vi "Display.vi"(8 "error in":errorcluster, 11 "Input (String) in":refnum<class "Custom - Input (String).lvclass">) -> (0 "error out":errorcluster, 3 "Input (String) out":refnum<class "Custom - Input (String).lvclass">)   [LabVIEW 2021, in "Pop-Up.lvlib" / "Custom - Input (String).lvclass"]
doc: "This vi will display the input pop up waiting for a type string input from the user while displaying a custom graphic to the user.\n\n<b>Code Developed By:</b> +\nDaniel Coons +\nhttps://github.com/danielcoons/tsc-pop-up"
uses:
  Custom - Input (String).lvclass
  C:/Development/Open Source/tsc-pop-up/Popup/Popup.lvclass
  Custom - Input (String).lvclass/Custom - Input (String).ctl
  Popup/Popup.lvclass/Popup.ctl
  Popup/Data Member Access/Read Theme.vi
  Theme/Theme.lvclass
  Popup/Popup.lvclass
  user32.dll
panel:
  out "header":bool
  in  "OK":bool
  in  "Input":string
  out "Input value out":string
  out "2D Picture":picture
  out "Message":string
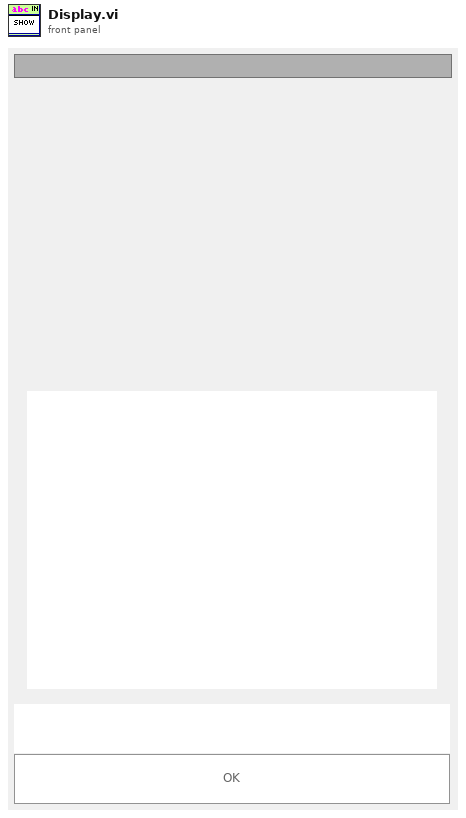
[diagram p1: front panel]
types:
  T1 = typedef "LVPoint32TypeDef.ctl" = cluster{"Horizontal":i32, "Vertical":i32}
  T2 = typedef "LVPositionTypeDef.ctl" = cluster{"Left":i32, "Top":i32}
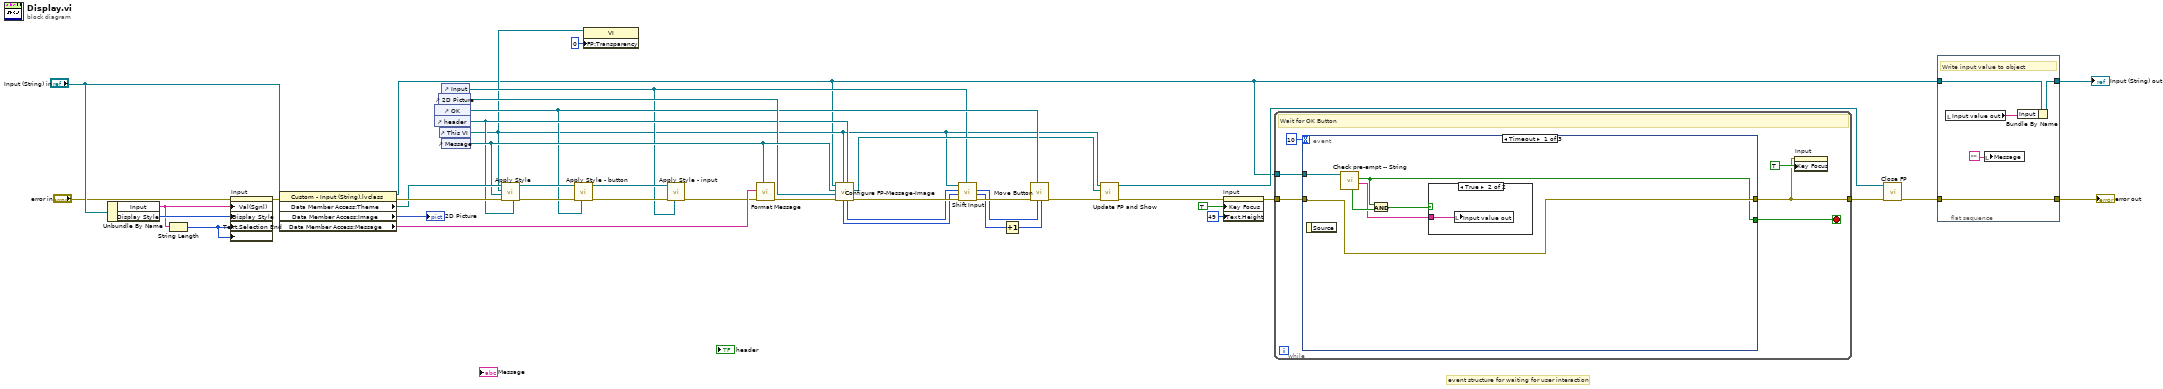
[diagram p0: block diagram]
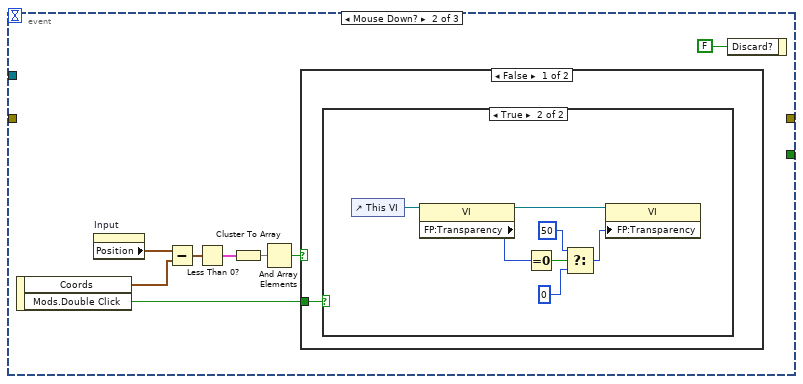
[diagram p3: hidden frame]
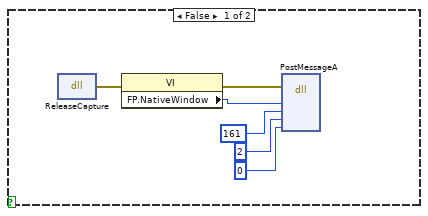
[diagram p4: hidden frame]
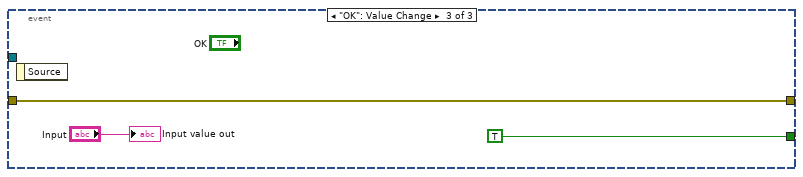
[diagram p6: hidden frame]
diagram:
  # "event structure for waiting for user interaction"
  n1 = Unbundle By Name("Input (String) in") -> ("Input"=w8:string, "Display Style"=w9:u32)
  n2 = String Length(string=w8) -> (length=w7:i32)
  n3 = property on="Input" class="Str"(error in="error in", "Val(Sgnl)"=w8, "Display Style"=w9, "Text.Selection End"=w7, "Text.Selection Start"=w7) -> (error out=w38:errorcluster)  [unwired: 1 in, 1 out]
  n4 = property class="Custom - Input (String).lvclass"(reference="Input (String) in", error in=w38) -> (reference out=w1:refnum<class "Custom - Input (String).lvclass">, error out=w37:errorcluster, "Data Member Access:Theme"=w27:refnum<class "Theme.lvclass">, "Data Member Access:Image"=→"2D Picture":picture, "Data Member Access:Message"=w29:string)
  n5 = control-ref of="OK"() -> (w14:refnum<vi>)
  n6 = control-ref of="header"() -> (w20:refnum<vi>)
  n7 = control-ref of="2D Picture"() -> (w21:refnum<vi>)
  n8 = control-ref of="This VI"() -> (w2:refnum<vi>)
  n9 = control-ref of="Input"() -> (w6:refnum<vi>)
  n10 = control-ref of="Message"() -> (w22:refnum<vi>)
  n11 = call "Apply Style.vi"("header ref"=w20, "error in"=w37, "message ref"=w22, "pop up ref"=w2, "Theme in"=w27) -> ("error out"=w28:errorcluster, "Theme out"=w25:refnum<class "Theme.lvclass">)  [unwired: 5 in]
  n12 = call "Apply Style - button.vi"("button ref"=w14, "error in"=w28, "Theme in"=w25) -> ("error out"=w26:errorcluster, "Theme out"=w23:refnum<class "Theme.lvclass">)  [unwired: 7 in]
  n13 = property on="Property Node" class="VI"(reference=w2, "FP:Transparency"=u8 0 ("Front Panel Window:Transparency")) -> ()  [unwired: 1 in, 2 out]
  n14 = call "Apply Style - input.vi"("input ref"=w6, "error in (no error)"=w26, "Theme in"=w23) -> ("error out"=w24:errorcluster)  [unwired: 7 in, 1 out]
  n15 = call "Format Message.vi"("formatted string"=w22, "error in"=w24, "String Input"=w29) -> ("error out"=w30:errorcluster)  [unwired: 7 in, 1 out]
  n16 = call "Configure FP-Message-Image.vi"("header ref"=w20, "Pop Up ref"=w2, "error in (no error)"=w30, "Image ref"=w21, "Message ref"=w22, "Popup in"=w1) -> ("error out"=w19:errorcluster, "Panel Ref"=w12:refnum<vi>, "Panel Width"=w17:i32, "Panel Height"=w16:i32)  [unwired: 1 in, 1 out]
  n17 = call "Shift Input.vi"("Control"=w6, "Error In"=w19, "Panel Height"=w16, "Panel Width"=w17, "Pop Up ref"=w2) -> ("Error Out"=w18:errorcluster, "Panel Height out"=w11:i32, "Panel Width out"=w13:i32)  [unwired: 4 in]
  n18 = Increment(x=w11) -> (x+1=w10:i32)
  n19 = call "Move Button.vi"("Panel Height"=w10, "Panel Width"=w13, "Button"=w14, "error in"=w18) -> ("error out"=w15:errorcluster)  [unwired: 6 in, 1 out]
  n20 = call "Update FP and Show.vi"("error in (no error)"=w15, "Panel Ref"=w12, "VI in"=w2) -> ("error out"=w34:errorcluster, "VI out"=w4:refnum<vi>)  [unwired: 7 in]
  n21 = property on="Input" class="Str"(error in=w34, "Key Focus"=TRUE, "Text.Height"=u32 49 ("Text.Size:Height")) -> (error out=w33:errorcluster)  [unwired: 1 in, 1 out]
  n22 = while {
    tunnel: w33 -> [w48]
    tunnel: [w43] -> w36
    tunnel: w1 -> [w45]
    stop <- w47 stop-if-true
    # "Wait for OK Button"
    n23 = event shown="[0] Timeout" {
      selector: _ -> [_ _ _]
      dyn-events: _ -> [_ _ _]
      timeout: 10 -> [_ _ _]
      tunnel: w48 -> [w50 _ w80]
      tunnel: [w50 _ w80] -> w43
      tunnel: [w49 _ TRUE] -> w47
      tunnel: w45 -> [w51 _ _]
      event Timeout {
        n24 = event-data() -> ()  [unwired: 1 in, 1 out]
        n25 = call "Check pre-empt -- String.vi"("_Popup in"=w51) -> ("Value?"=w52:string, "Pre-empted?"=w49:bool, "Type Match?"=w54:bool)  [unwired: 7 in, 1 out]
        n26 = Compound Arithmetic op=AND(w49, w54) -> (w53:bool)
        n27 = case shown="True" w53 {
          tunnel: w52 -> [_ w55]
          frame False {
          }
          frame True {
            n28 = local write "Input value out"(w55) -> ()
          }
        }
      }
      event Mouse Down? {
        n29 = event-data() -> ("Coords"=w57:T1, "Mods.Double Click"=w56:bool)  [unwired: 1 in]
        n30 = property on="Input" class="Str"() -> ("Position"=w58:T2)  [unwired: 2 in, 2 out]
        n31 = Subtract(x=w58, y=w57) -> (x-y=w59:T2)
        n32 = Less Than 0?(x=w59) -> (x < 0?=w60:cluster{"Left":bool, "Top":bool})
        n33 = Cluster To Array(cluster=w60) -> (array=w61:bool[])
        n34 = And Array Elements(Boolean array=w61) -> (logical AND=w62:bool)
        n35 = case shown="False" w62 {
          tunnel: w56 -> [w64 _]
          frame False {
            n36 = case shown="True" w64 {
              frame False {
                n37 = dll-call lib="user32.dll" fn="ReleaseCapture"() -> (error out=w68:errorcluster)  [unwired: 4 in, 1 out]
                n38 = property class="VI"(error in=w68) -> (error out=w69:errorcluster, "FP.NativeWindow"=w70:u64)  [unwired: 1 in, 1 out]
                n39 = dll-call lib="user32.dll" fn="PostMessageA"(error in=w69, "hWnd"=w70, "Msg"=161, "wParam"=2, "lParam"=0) -> ()  [unwired: 7 in, 2 out]
              }
              frame True {
                n40 = control-ref of="This VI"() -> (w77:refnum<vi>)
                n41 = property class="VI"(reference=w77) -> (reference out=w75:refnum<vi>, "FP:Transparency"=w76:u8)  [unwired: 1 in, 1 out]
                n42 = Equal To 0?(x=w76) -> (x = 0?=w74:bool)
                n43 = Select(t=u8 50, s=w74, f=u8 0) -> (s? t:f=w73:u8)
                n44 = property class="VI"(reference=w75, "FP:Transparency"=w73) -> ()  [unwired: 1 in, 2 out]
              }
            }
          }
          frame True {
          }
        }
        n45 = event-data("Discard?"=FALSE) -> ()  [unwired: 1 in, 1 out]
      }
      event "OK": Value Change {
        n46 = event-data() -> ()  [unwired: 1 in, 1 out]
        "Input value out" <- "Input"
      }
    }
    n47 = property on="Input" class="Str"(error in=w43, "Key Focus"=TRUE) -> ()  [unwired: 1 in, 2 out]
  }
  n48 = call "Close FP.vi"("error in (no error)"=w36, "VI in"=w4) -> ("error out"=w35:errorcluster)  [unwired: 9 in]
  n49 = flat-sequence {
    tunnel: w35 -> [w85]
    tunnel: [w85] -> w39
    tunnel: w1 -> [w84]
    tunnel: [w83] -> w40
    frame #0 {
      # "Write input value to object"
      n50 = local read "Input value out"() -> (w82:string)
      n51 = local write "Message"("" ("Message")) -> ()
      n52 = Bundle By Name(cluster=w84, "Input"=w82) -> (w83:refnum<class "Custom - Input (String).lvclass">)
    }
  }
  "error out" <- w39
  "Input (String) out" <- w40
